vi "側推主程式(c58).vi"() -> ()   [LabVIEW 2021]
uses:
  <vilib>/Analysis/baseanly.llb/Mean (DBL).vi
  <vilib>/Analysis/NI_AALBase.lvlib
panel:
  out "Save A":bool
  out "Save 9":bool
  out "Save 7":bool
  out "A stop":bool
  out "A run":bool
  out "R stop":bool
  out "R run":bool
  out "AO stop":bool
  out "AO run":bool
  in  "Tab Control":T1(tab)
  in  "Tab Control 2":enum32{"循環加載", "線性加載", "定值加載"}(tab)
  out "AO Chart basic_cyc":dbl(graph)
  out "XY end":dbl=1.0
  out "basic end":dbl
  in  "AO stop\n(F時連續cyc)\n(T時停止AO)":bool
  out "t'(目前加載次數)":dbl
  out "T為完成加載":bool
  out "dt(目前歷時)":dbl
  out "duration":dbl
  in  "number of cyc":dbl
  out "AO Chart y_cyc":dbl(graph)
  out "AO Chart x_cyc":dbl(graph)
  in  "basic":dbl
  in  "cyc平移調整y":dbl
  in  "cyc震幅調整y":dbl
  in  "(basic+震幅)\ncyc平移調整x":dbl
  in  "cyc震幅調整x":dbl
  in  "fre(Hz)":dbl
  in  "milliseconds to (設定0)":u32
  in  "線性電壓斜率y":dbl
  in  "線性電壓斜率x":dbl
  out "線性加載 Chart":dynamicdata(graph)
  in  "線性加載初值 Y":dbl
  in  "線性加載初值 X":dbl
  in  "線性加載 basic":dbl
  out "非循環歷時 2":dbl
  out "線性加載\nbasic end":dbl
  in  "線性加載\n(F為連續)\n(T為停止)":bool
  out "XY end":dbl=1.0
  out "EP_X":dbl
  out "EP_Y":dbl
  out "EP_B":dbl
  out "非循環歷時":dbl
  out "定值加載\nbasic end":dbl
  out "XY end":dbl=1.0
  in  "定值加載\n(F為連續)\n(T為停止)":bool
  in  "定值加載 Y":dbl
  in  "定值加載 X":dbl
  in  "定值加載 basic":dbl
  out "定值加載 Chart":dynamicdata(graph)
  in  "線性加載\n(T為X加載)\n(F為Y加載)":bool
  in  "非循環加載\n(T為定值加載)\n(F為線性加載)":bool
  in  "循環加載\n(T為循環加載)\n(F為非循環加載)":bool
  in  "T為開始側推\nF為等待下一步指令\n(一開始先T)":bool
  out "Waveform Chart S7":dynamicdata(graph)
  in  "rate S7":dbl=1000.0
  in  "number of samples S7":i32=100
  out "Waveform Chart S9":dynamicdata(graph)
  in  "number of samples S9":i32=100
  in  "rate S9":dbl=1000.0
  in  "Enable S7":bool=TRUE caption="Enable"
  in  "Filename S7":path=path "test.lvm" caption="Filename"
  in  "Enable S9":bool=TRUE caption="Enable"
  in  "Filename S9":path=path "test.lvm" caption="Filename"
  in  "F 為\n開始 reading\n(AO is continue)":bool
  out "ACC紀錄中":bool
  out "Waveform Graph ACC":dynamicdata(graph)
  in  "number of samples":i32=2000
  in  "rate":dbl=20000.0
  in  "Enable":bool=TRUE
  in  "Filename":path=path "test.lvm"
  in  "Boolean\n(T為開始記讀)\n(F為停止記讀)\n(T後請手動調成F，避免重複執行)":bool
  out "Waveform Chart 角度cos_Y 3":dbl(graph)
  out "Waveform Chart LDT_X real":dynamicdata(graph)
  out "Waveform Chart load real 2":dynamicdata(graph)
  out "Waveform Chart 樁頭dis_X":dbl(graph)
  in  "LDT20係數":dbl
  in  "LDT20初值":dbl
  in  "LDT29係數":dbl
  in  "LDT29初值":dbl
  in  "LDT11初值":dbl
  in  "LDT11係數":dbl
  in  "LDT12係數":dbl
  in  "LDT12初值":dbl
  in  "PPT_B係數":dbl
  in  "PPT_B初值":dbl
  in  "PPT_C係數":dbl
  in  "PPT_C初值":dbl
  in  "PPT_E係數":dbl
  in  "PPT_E初值":dbl
  in  "PPT_F係數":dbl
  in  "PPT_F初值":dbl
  out "Waveform Chart PPT real":dynamicdata(graph)
  out "Waveform Chart load real":dynamicdata(graph)
  in  "load_X初值":dbl
  in  "load_Y初值":dbl
  in  "load_X係數":dbl
  in  "load_Y係數":dbl
  out "LDT20 real":dbl
  out "LDT29 real":dbl
  out "LDT12 real":dbl
  out "LDT11 real":dbl
  in  "LDT_X間距\n(cm)_3-4cm":dbl
  in  "LDT_Y間距\n(cm)_5.2cm":dbl
  out "LDT_Y斜率":dbl
  out "LDT_X斜率":dbl
  out "樁頭位移_X(cm)":dbl
  out "樁頭位移_Y(cm)":dbl
  in  "樁頭離\n下側LDT距_X\n(cm)":dbl
  in  "樁頭離\n下側LDT距_Y\n(cm)":dbl
  out "樁角度_Y_tan":dbl
  out "樁角度_X_tan":dbl
  out "Waveform Chart 樁頭dis_Y":dbl(graph)
  out "Waveform Chart 角度tan_Y":dbl(graph)
  out "Waveform Chart 角度tan_X":dbl(graph)
  out "樁角度_Y_cos":dbl
  out "Waveform Chart 角度cos_X":dbl(graph)
  out "樁角度_X_cos":dbl
  out "mean_load_Y":dbl format="%0.2f"
  out "mean_load_X":dbl format="%0.2f"
  out "Waveform Chart LDT_Y real 2":dynamicdata(graph)
  out "Waveform Chart LDT_Y real":dynamicdata(graph)
  out "Waveform Chart LDT_X real 2":dynamicdata(graph)
  # "AO"
  # "Read"
  # "ACC"
  # "資料擷取比\n電壓輸出快3s"
  # "循環"
  # "basic = XY\n完成反覆側推後\n側推力平衡"
  # "線性\n分X、Y向"
  # "定值"
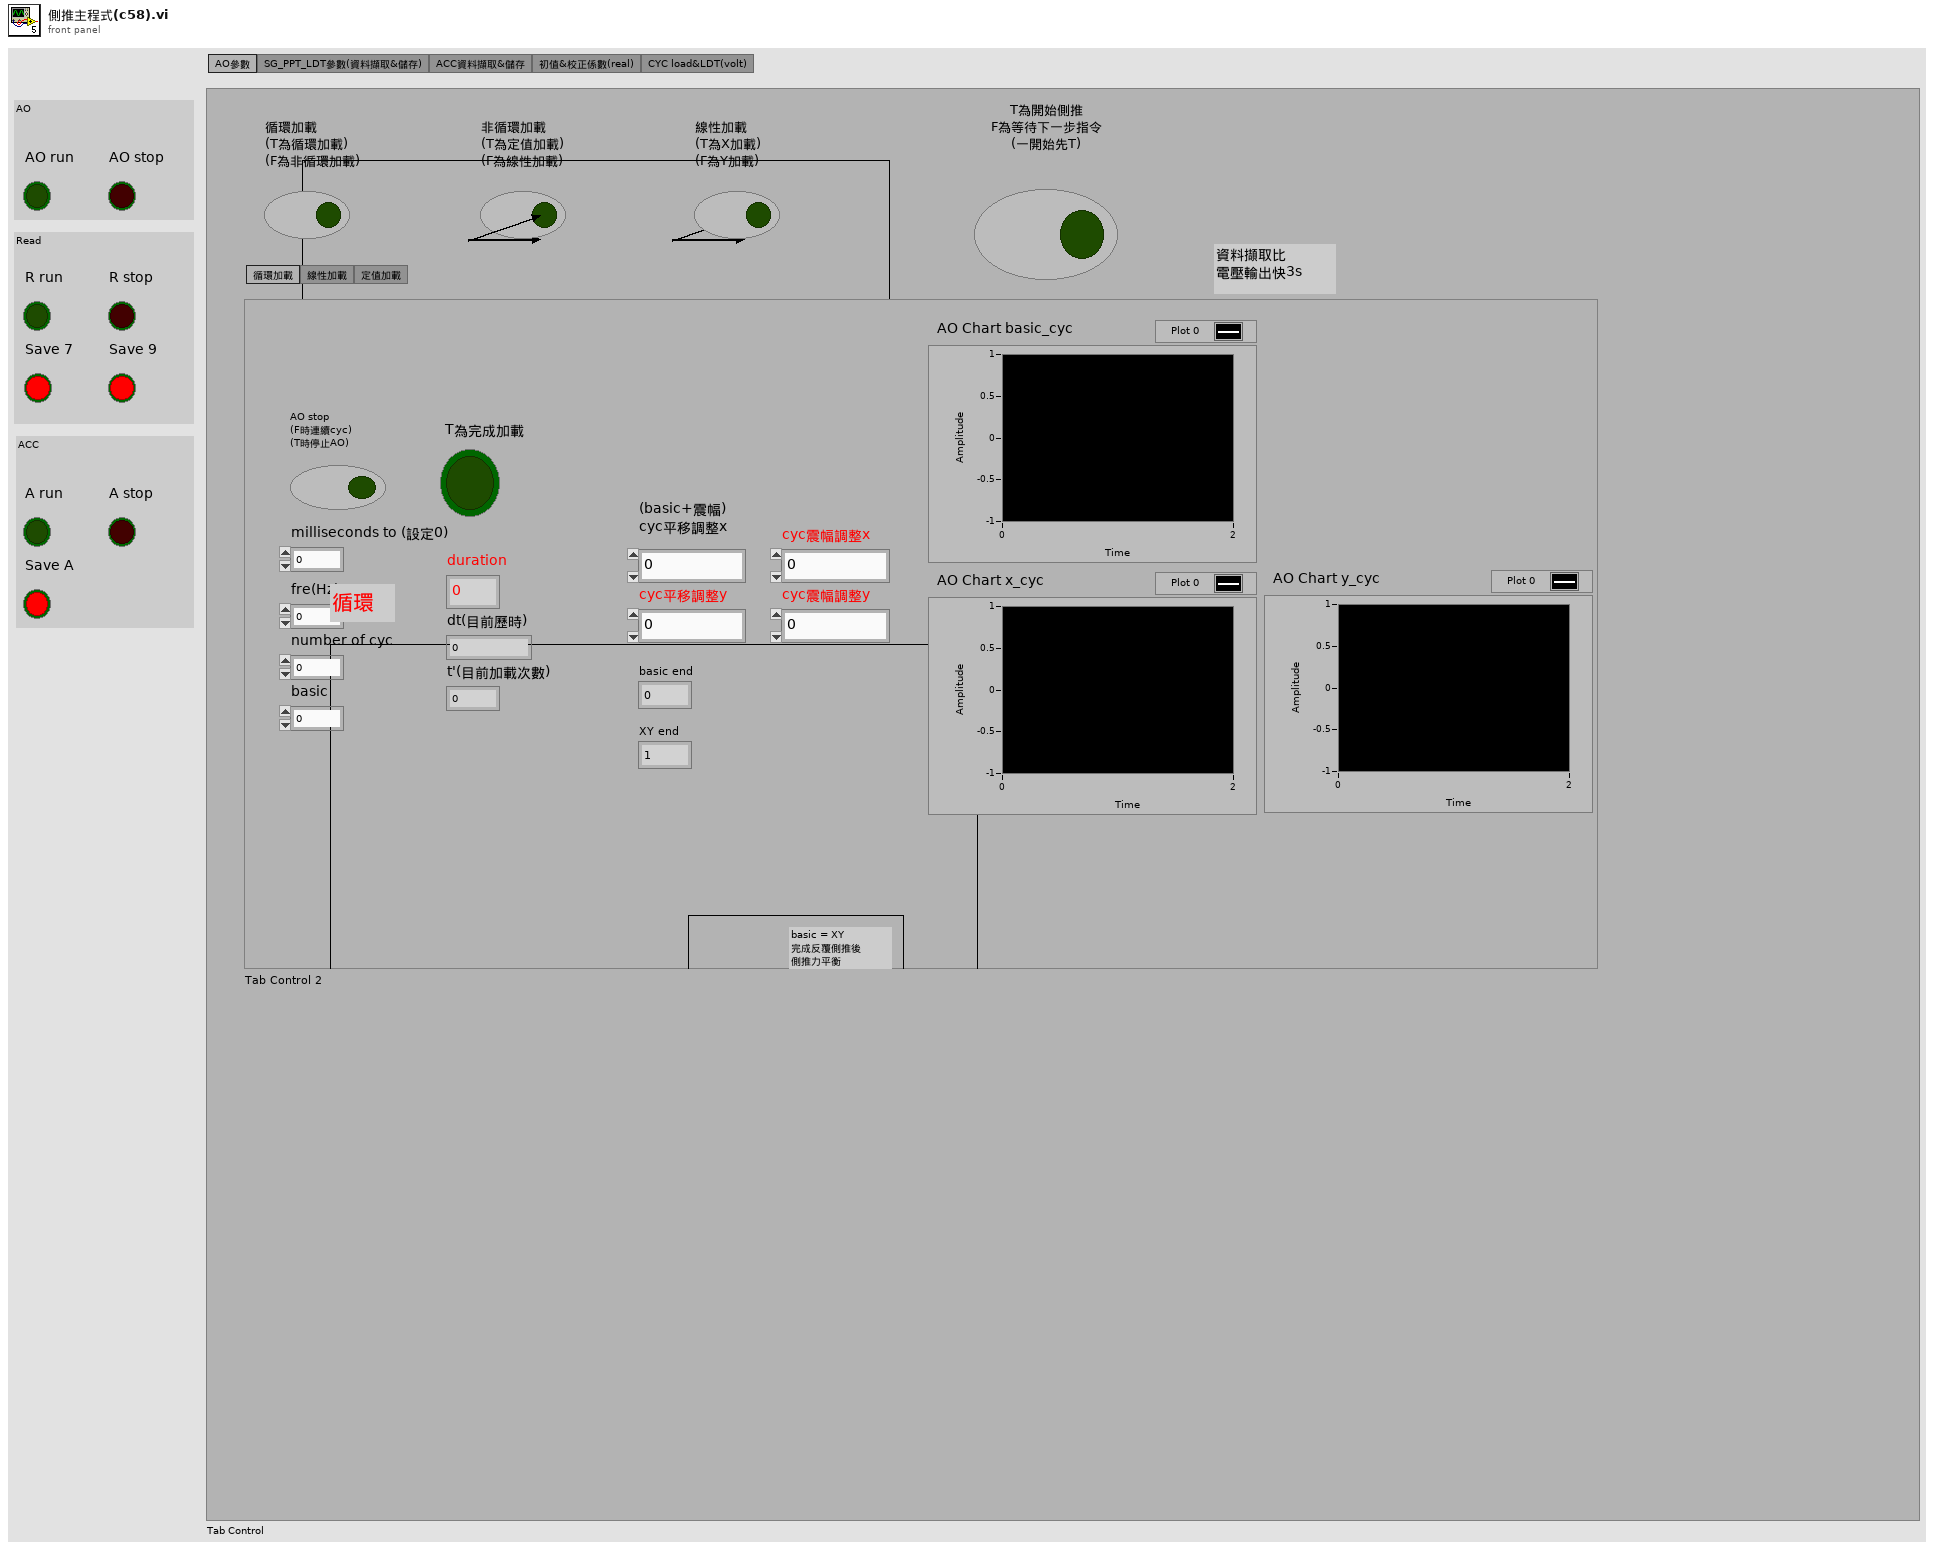
[diagram p1: front panel]
types:
  T1 = enum32{"AO參數", "SG_PPT_LDT參數(資料擷取&儲存)", "ACC資料擷取&儲存", "初值&校正係數(real)", "CYC load&LDT(volt)"}
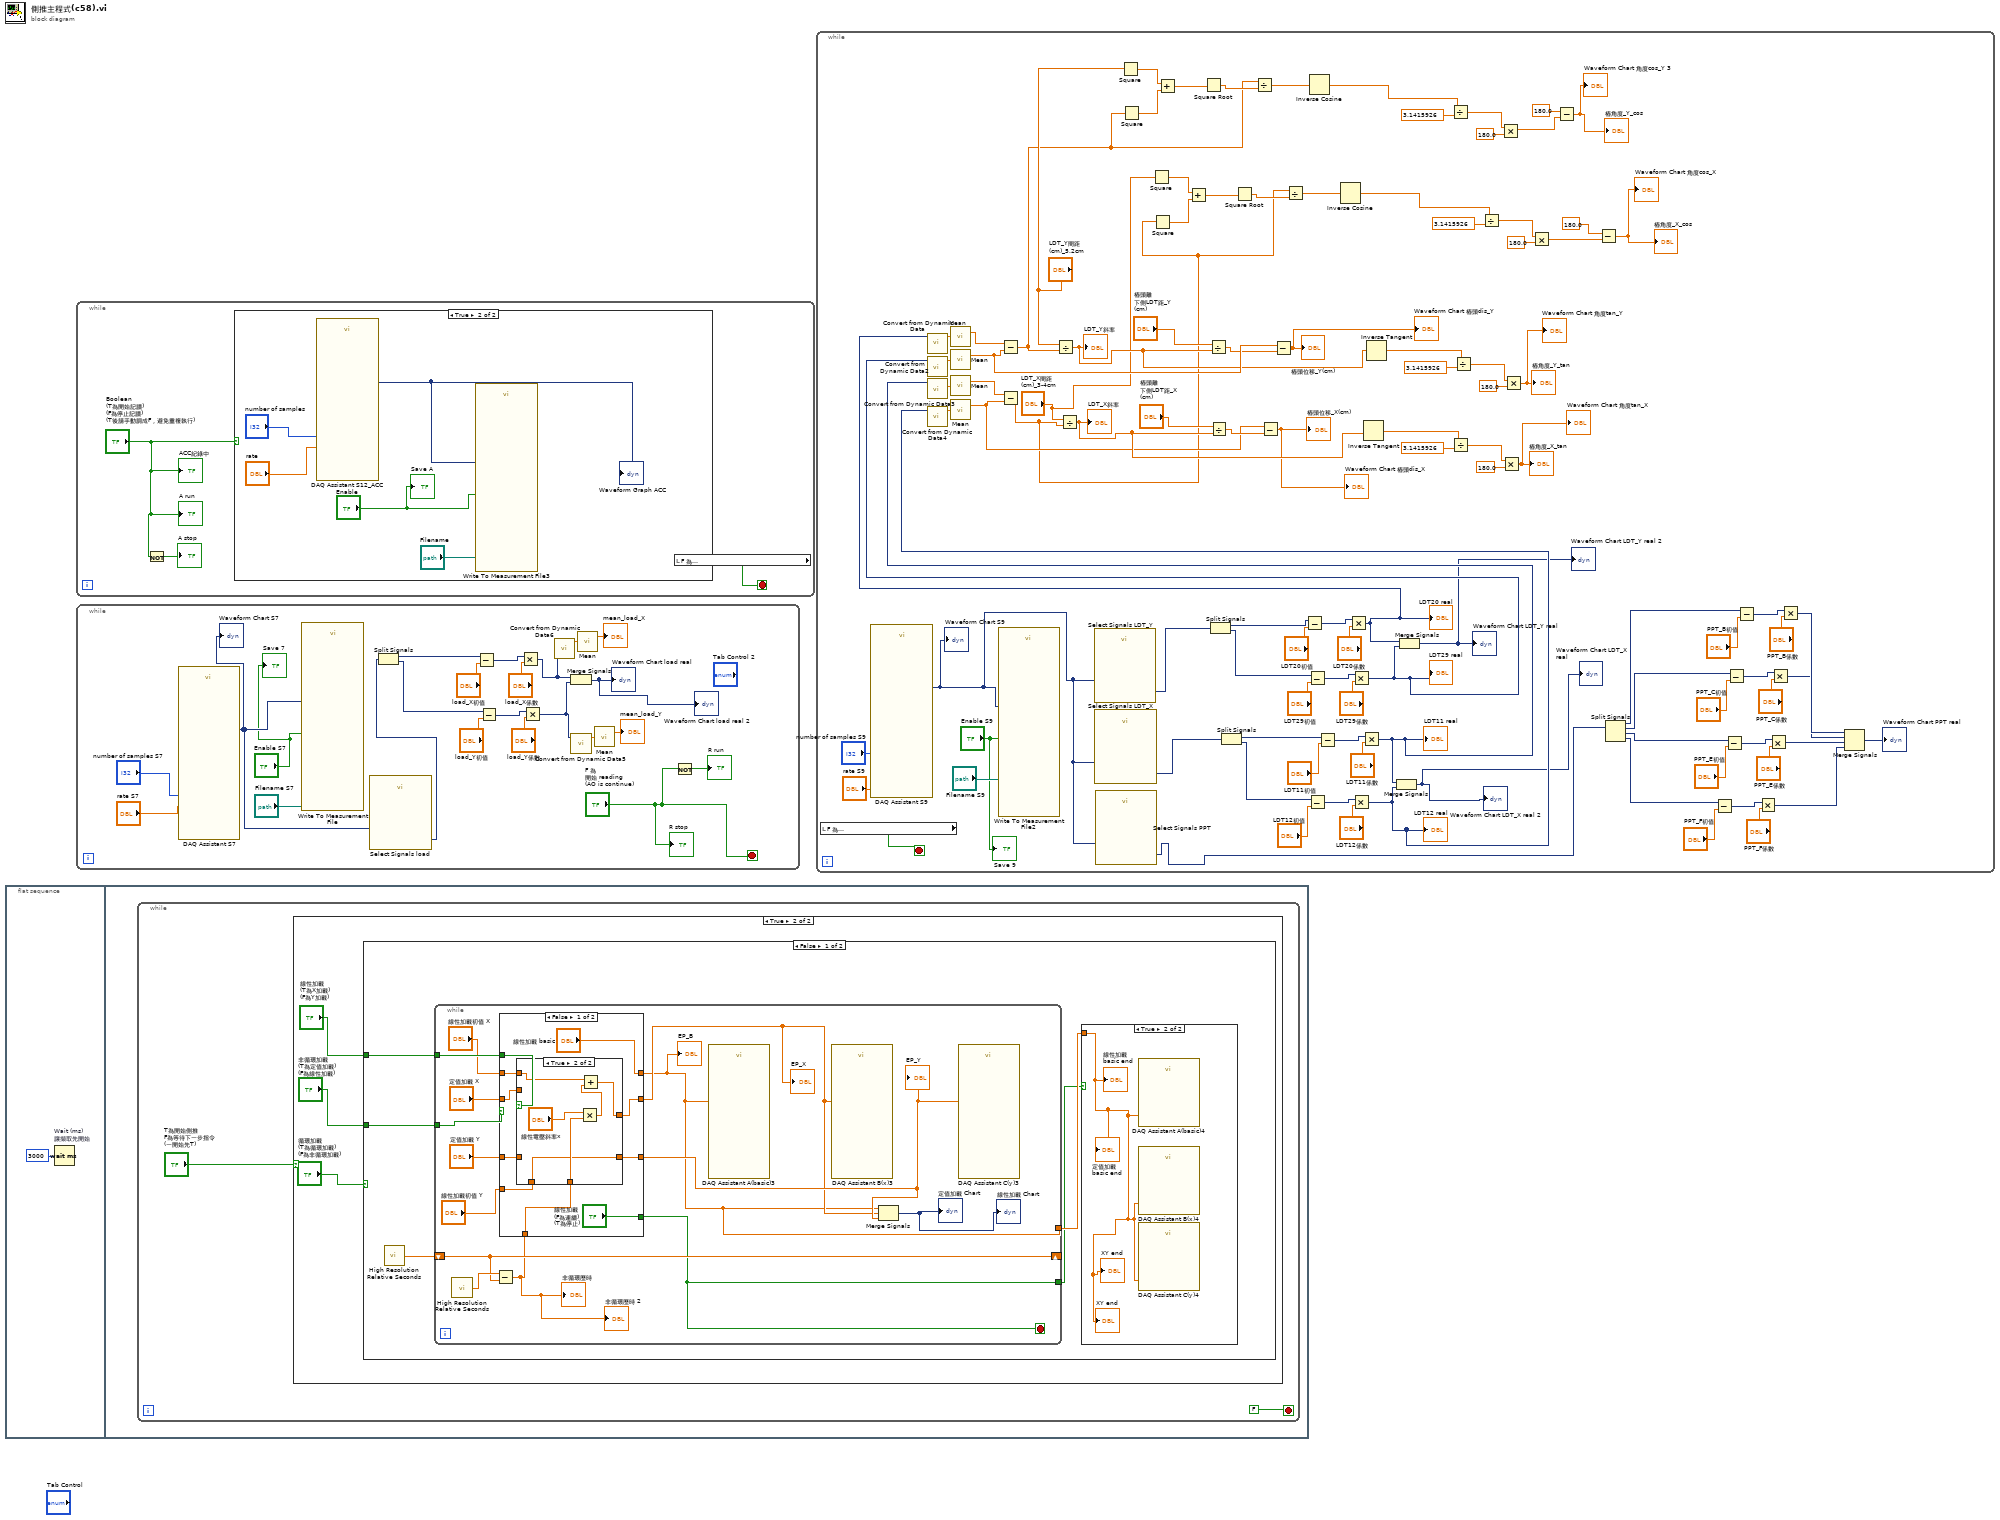
[diagram p0: block diagram]
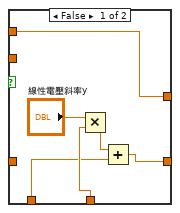
[diagram p5: hidden frame]
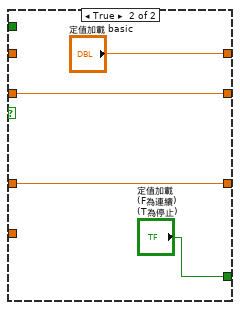
[diagram p6: hidden frame]
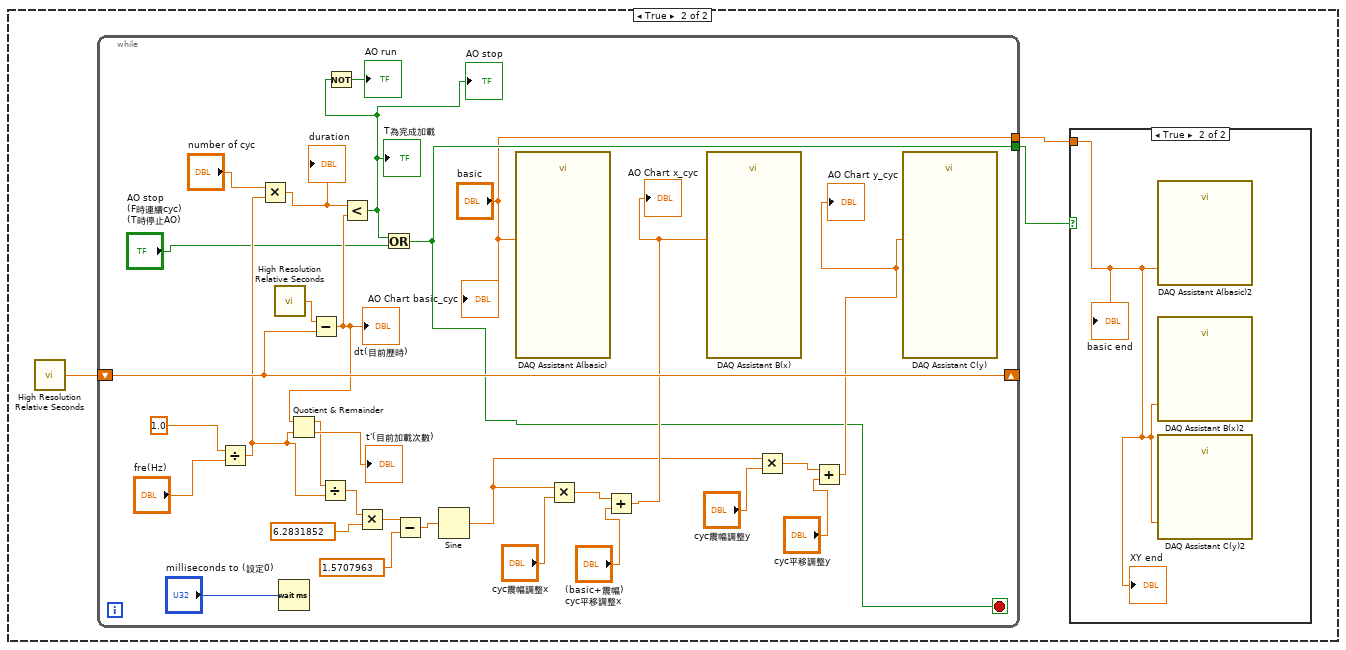
[diagram p7: hidden frame]
diagram:
  n1 = flat-sequence {
    frame #0 {
      n2 = Wait (ms) "Wait (ms)\n讓擷取先開始"(milliseconds to wait=u32 3000) -> ()  [unwired: 1 out]
    }
    frame #1 {
      n3 = while {
        stop <- FALSE stop-if-true
        n4 = case shown="True" "T為開始側推\nF為等待下一步指令\n(一開始先T)" {
          frame False {
          }
          frame True {
            n5 = case shown="False" "循環加載\n(T為循環加載)\n(F為非循環加載)" {
              tunnel: "非循環加載\n(T為定值加載)\n(F為線性加載)" -> [w8 _]
              tunnel: "線性加載\n(T為X加載)\n(F為Y加載)" -> [w7 _]
              frame False {
                n6 = call <vilib>:"High Resolution Relative Seconds.vi"() -> ("relative seconds"=w10:dbl)
                n7 = while {
                  tunnel: [w13] -> w11
                  shift-right: [w25] -> _
                  shift-left: w10 -> [w25]
                  tunnel: [w15] -> w9
                  tunnel: w8 -> [w24]
                  tunnel: w7 -> [w20]
                  stop <- w15 stop-if-true
                  n8 = call <vilib>:"High Resolution Relative Seconds.vi"() -> ("relative seconds"=w26:dbl)
                  n9 = Subtract(x=w26, y=w25) -> (x-y=w16:dbl)
                  "非循環歷時" <- w16
                  "非循環歷時 2" <- w16
                  n10 = case shown="False" w24 {
                    tunnel: "定值加載 X" -> [w31 w52]
                    tunnel: [w33 w52] -> w14
                    tunnel: "定值加載 Y" -> [w34 w51]
                    tunnel: [w32 w51] -> w21
                    tunnel: w16 -> [w36 _]
                    tunnel: w20 -> [w35 _]
                    tunnel: "線性加載初值 X" -> [w30 _]
                    tunnel: "線性加載初值 Y" -> [w29 _]
                    tunnel: ["線性加載 basic" "定值加載 basic"] -> w13
                    tunnel: ["線性加載\n(F為連續)\n(T為停止)" "定值加載\n(F為連續)\n(T為停止)"] -> w15
                    frame False {
                      n11 = case shown="True" w35 {
                        tunnel: w36 -> [w41 w47]
                        tunnel: [w40 w43] -> w33
                        tunnel: w34 -> [_ _]
                        tunnel: [w37 w46] -> w32
                        tunnel: w31 -> [_ _]
                        tunnel: w30 -> [w40 w45]
                        tunnel: w29 -> [w38 w46]
                        frame False {
                          n12 = Multiply(x="線性電壓斜率y", y=w41) -> (x*y=w39:dbl)
                          n13 = Add(x=w39, y=w38) -> (x+y=w37:dbl)
                        }
                        frame True {
                          n14 = Multiply(x="線性電壓斜率x", y=w47) -> (x*y=w44:dbl)
                          n15 = Add(x=w45, y=w44) -> (x+y=w43:dbl)
                        }
                      }
                    }
                    frame True {
                    }
                  }
                  "EP_Y" <- w21
                  "EP_X" <- w14
                  "EP_B" <- w13
                  n16 = call "DAQ Assistant A(basic)3"("data"=w13) -> ()  [unwired: 17 in, 2 out]
                  n17 = call "DAQ Assistant B(x)3"("data"=w14) -> ()  [unwired: 17 in, 2 out]
                  n18 = Merge Signals(w13, w14, w21) -> (→"定值加載 Chart" →"線性加載 Chart":dynamicdata)
                  n19 = call "DAQ Assistant C(y)3"("data"=w21) -> ()  [unwired: 17 in, 2 out]
                }
                n20 = case shown="True" w9 {
                  tunnel: w11 -> [_ w12]
                  frame False {
                  }
                  frame True {
                    n21 = call "DAQ Assistant A(basic)4"("data"=w12) -> ()  [unwired: 17 in, 2 out]
                    n22 = call "DAQ Assistant B(x)4"("data"=w12) -> ()  [unwired: 17 in, 2 out]
                    n23 = call "DAQ Assistant C(y)4"("data"=w12) -> ()  [unwired: 17 in, 2 out]
                    "定值加載\nbasic end" <- w12
                    "XY end" <- w12
                    "線性加載\nbasic end" <- w12
                    "XY end" <- w12
                  }
                }
              }
              frame True {
                n24 = call <vilib>:"High Resolution Relative Seconds.vi"() -> ("relative seconds"=w55:dbl)
                n25 = while {
                  shift-right: [w85] -> _
                  shift-left: w55 -> [w85]
                  tunnel: [w64] -> w54
                  tunnel: ["basic"] -> w53
                  stop <- w64 stop-if-true
                  n26 = Divide(x=1.0, y="fre(Hz)") -> (x/y=w68:dbl)
                  n27 = Multiply(x="number of cyc", y=w68) -> (x*y=w67:dbl)
                  "duration" <- w67
                  n28 = call <vilib>:"High Resolution Relative Seconds.vi"() -> ("relative seconds"=w86:dbl)
                  n29 = Wait (ms)(milliseconds to wait="milliseconds to (設定0)") -> ()  [unwired: 1 out]
                  n30 = Subtract(x=w86, y=w85) -> (x-y=w66:dbl)
                  "dt(目前歷時)" <- w66
                  n31 = Quotient & Remainder(x=w66, y=w68) -> (x-y*floor(x/y)=w81:dbl, floor(x/y)=→"t'(目前加載次數)":dbl)
                  n32 = Divide(x=w81, y=w68) -> (x/y=w78:dbl)
                  n33 = Less?(x=w67, y=w66) -> (x < y?=w58:bool)
                  "T為完成加載" <- w58
                  "AO stop" <- w58
                  n34 = Not(x=w58) -> (.not. x?=→"AO run":bool)
                  n35 = Multiply(x=w78, y=6.2831852) -> (x*y=w61:dbl)
                  n36 = Or(x=w58, y="AO stop\n(F時連續cyc)\n(T時停止AO)") -> (x .or. y?=w64:bool)
                  n37 = Subtract(x=w61, y=1.5707963) -> (x-y=w60:dbl)
                  n38 = Sine(x=w60) -> (sin(x)=w59:dbl)
                  n39 = call "DAQ Assistant A(basic)"("data"="basic") -> ()  [unwired: 17 in, 2 out]
                  n40 = Multiply(x=w59, y="cyc震幅調整x") -> (x*y=w76:dbl)
                  n41 = Add(x=w76, y="(basic+震幅)\ncyc平移調整x") -> (x+y=w71:dbl)
                  "AO Chart x_cyc" <- w71
                  n42 = call "DAQ Assistant B(x)"("data"=w71) -> ()  [unwired: 17 in, 2 out]
                  n43 = Multiply(x=w59, y="cyc震幅調整y") -> (x*y=w73:dbl)
                  n44 = Add(x=w73, y="cyc平移調整y") -> (x+y=w70:dbl)
                  "AO Chart y_cyc" <- w70
                  n45 = call "DAQ Assistant C(y)"("data"=w70) -> ()  [unwired: 17 in, 2 out]
                  "AO Chart basic_cyc" <- "basic"
                }
                n46 = case shown="True" w54 {
                  tunnel: w53 -> [_ w56]
                  frame False {
                  }
                  frame True {
                    n47 = call "DAQ Assistant A(basic)2"("data"=w56) -> ()  [unwired: 17 in, 2 out]
                    n48 = call "DAQ Assistant B(x)2"("data"=w56) -> ()  [unwired: 17 in, 2 out]
                    n49 = call "DAQ Assistant C(y)2"("data"=w56) -> ()  [unwired: 17 in, 2 out]
                    "basic end" <- w56
                    "XY end" <- w56
                  }
                }
              }
            }
          }
        }
      }
    }
  }
  n50 = while {
    stop <- w89 stop-if-true
    n51 = Not(x="Boolean\n(T為開始記讀)\n(F為停止記讀)\n(T後請手動調成F，避免重複執行)") -> (.not. x?=→"A stop":bool)
    n52 = case shown="True" "Boolean\n(T為開始記讀)\n(F為停止記讀)\n(T後請手動調成F，避免重複執行)" {
      frame False {
      }
      frame True {
        n53 = call "DAQ Assistant S12_ACC"("rate"="rate", "number of samples"="number of samples") -> ("data"=w92:dynamicdata)  [unwired: 15 in, 2 out]
        "Waveform Graph ACC" <- w92
        n54 = call "Write To Measurement File3"("Signals"=w92, "Enable"="Enable", "Filename"="Filename") -> ()  [unwired: 14 in, 3 out]
        "Save A" <- "Enable"
      }
    }
    n55 = local read "F 為\n開始 reading\n(AO is continue)"() -> (w89:bool)
    "ACC紀錄中" <- "Boolean\n(T為開始記讀)\n(F為停止記讀)\n(T後請手動調成F，避免重複執行)"
    "A run" <- "Boolean\n(T為開始記讀)\n(F為停止記讀)\n(T後請手動調成F，避免重複執行)"
  }
  n56 = while {
    stop <- "F 為\n開始 reading\n(AO is continue)" stop-if-true
    n57 = call "DAQ Assistant S7"("rate"="rate S7", "number of samples"="number of samples S7") -> ("data"=w105:dynamicdata)  [unwired: 14 in, 3 out]
    "Waveform Chart S7" <- w105
    n58 = call "Write To Measurement File"("Signals"=w105, "Enable"="Enable S7", "Filename"="Filename S7") -> ()  [unwired: 14 in, 3 out]
    n59 = call "Select Signals load"("Signals"=w105) -> ("Signal Out"=w108:dynamicdata)  [unwired: 9 in, 1 out]
    n60 = Split Signals(w108) -> (w107:dynamicdata, w106:dynamicdata)  [unwired: 2 in]
    n61 = Subtract(x=w107, y="load_X初值") -> (x-y=w114:dynamicdata)
    n62 = Subtract(x=w106, y="load_Y初值") -> (x-y=w111:dynamicdata)
    n63 = Multiply(x=w114, y="load_X係數") -> (x*y=w100:dynamicdata)
    n64 = Multiply(x=w111, y="load_Y係數") -> (x*y=w104:dynamicdata)
    n65 = call "Convert from Dynamic Data6"("Dynamic Data Type"=w100) -> ("Array"=w99:dbl[])  [unwired: 3 in]
    n66 = Merge Signals(w100, w104) -> (→"Waveform Chart load real" →"Waveform Chart load real 2":dynamicdata)
    n67 = call "Convert from Dynamic Data5"("Dynamic Data Type"=w104) -> ("Array"=w103:dbl[])  [unwired: 3 in]
    n68 = call-poly <vilib>:"Mean.vi"("X"=w99) -> ("mean"=→"mean_load_X":dbl)  [unwired: 1 out]
    n69 = call-poly <vilib>:"Mean.vi"("X"=w103) -> ("mean"=→"mean_load_Y":dbl)  [unwired: 1 out]
    n70 = Not(x="F 為\n開始 reading\n(AO is continue)") -> (.not. x?=→"R run":bool)
    "R stop" <- "F 為\n開始 reading\n(AO is continue)"
    "Save 7" <- "Enable S7"
  }
  n71 = while {
    stop <- w127 stop-if-true
    n72 = local read "F 為\n開始 reading\n(AO is continue)"() -> (w127:bool)
    n73 = call "DAQ Assistant S9"("rate"="rate S9", "number of samples"="number of samples S9") -> ("data"=w220:dynamicdata)  [unwired: 14 in, 3 out]
    "Waveform Chart S9" <- w220
    n74 = call "Write To Measurement File2"("Signals"=w220, "Enable"="Enable S9", "Filename"="Filename S9") -> ()  [unwired: 14 in, 3 out]
    n75 = call "Select Signals LDT_Y"("Signals"=w220) -> ("Signal Out"=w219:dynamicdata)  [unwired: 9 in, 1 out]
    n76 = call "Select Signals LDT_X"("Signals"=w220) -> ("Signal Out"=w208:dynamicdata)  [unwired: 9 in, 1 out]
    n77 = call "Select Signals PPT"("Signals"=w220) -> ("Signal Out"=w184:dynamicdata)  [unwired: 9 in, 1 out]
    n78 = Square(x="LDT_Y間距\n(cm)_5.2cm") -> (x^2=w149:dbl)
    n79 = Square(x="LDT_X間距\n(cm)_3-4cm") -> (x^2=w138:dbl)
    n80 = Split Signals(w219) -> (w216:dynamicdata, w211:dynamicdata)  [unwired: 2 in]
    n81 = Split Signals(w208) -> (w206:dynamicdata, w202:dynamicdata)  [unwired: 2 in]
    n82 = Subtract(x=w216, y="LDT20初值") -> (x-y=w218:dynamicdata)
    n83 = Subtract(x=w211, y="LDT29初值") -> (x-y=w214:dynamicdata)
    n84 = Subtract(x=w202, y="LDT12初值") -> (x-y=w205:dynamicdata)
    n85 = Subtract(x=w206, y="LDT11初值") -> (x-y=w210:dynamicdata)
    n86 = Multiply(x=w218, y="LDT20係數") -> (x*y=w179:dynamicdata)
    "LDT20 real" <- w179
    n87 = call "Convert from Dynamic Data"("Dynamic Data Type"=w179) -> ("Array"=w178:dbl[])  [unwired: 3 in]
    n88 = call-poly <vilib>:"Mean.vi"("X"=w178) -> ("mean"=w170:dbl)  [unwired: 1 out]
    n89 = Multiply(x=w214, y="LDT29係數") -> (x*y=w177:dynamicdata)
    "LDT29 real" <- w177
    n90 = call "Convert from Dynamic Data2"("Dynamic Data Type"=w177) -> ("Array"=w176:dbl[])  [unwired: 3 in]
    n91 = call-poly <vilib>:"Mean.vi"("X"=w176) -> ("mean"=w167:dbl)  [unwired: 1 out]
    n92 = Subtract(x=w170, y=w167) -> (x-y=w139:dbl)
    n93 = Divide(x="LDT_Y間距\n(cm)_5.2cm", y=w139) -> (x/y=w160:dbl)
    "LDT_Y斜率" <- w160
    n94 = Square(x=w139) -> (x^2=w148:dbl)
    n95 = Add(x=w149, y=w148) -> (x+y=w147:dbl)
    n96 = Square Root(x=w147) -> (sqrt(x)=w146:dbl)
    n97 = Divide(x="樁頭離\n下側LDT距_Y\n(cm)", y=w160) -> (x/y=w166:dbl)
    n98 = Divide(x=w139, y=w146) -> (x/y=w144:dbl)
    n99 = Subtract(x=w167, y=w166) -> (x-y=→"樁頭位移_Y(cm)" →"Waveform Chart 樁頭dis_Y":dbl)
    n100 = Inverse Cosine(1:w144) -> (0:w140:dbl)
    n101 = Multiply(x=w205, y="LDT12係數") -> (x*y=w173:dynamicdata)
    "LDT12 real" <- w173
    n102 = call "Convert from Dynamic Data4"("Dynamic Data Type"=w173) -> ("Array"=w172:dbl[])  [unwired: 3 in]
    n103 = call-poly <vilib>:"Mean.vi"("X"=w172) -> ("mean"=w151:dbl)  [unwired: 1 out]
    n104 = Multiply(x=w210, y="LDT11係數") -> (x*y=w175:dynamicdata)
    "LDT11 real" <- w175
    n105 = call "Convert from Dynamic Data3"("Dynamic Data Type"=w175) -> ("Array"=w174:dbl[])  [unwired: 3 in]
    n106 = call-poly <vilib>:"Mean.vi"("X"=w174) -> ("mean"=w171:dbl)  [unwired: 1 out]
    n107 = Subtract(x=w171, y=w151) -> (x-y=w128:dbl)
    n108 = Divide(x="LDT_X間距\n(cm)_3-4cm", y=w128) -> (x/y=w155:dbl)
    "LDT_X斜率" <- w155
    n109 = Square(x=w128) -> (x^2=w137:dbl)
    n110 = Add(x=w138, y=w137) -> (x+y=w136:dbl)
    n111 = Divide(x="樁頭離\n下側LDT距_X\n(cm)", y=w155) -> (x/y=w165:dbl)
    n112 = Square Root(x=w136) -> (sqrt(x)=w135:dbl)
    n113 = Subtract(x=w151, y=w165) -> (x-y=→"樁頭位移_X(cm)" →"Waveform Chart 樁頭dis_X":dbl)
    n114 = Divide(x=w128, y=w135) -> (x/y=w134:dbl)
    n115 = Inverse Cosine(1:w134) -> (0:w130:dbl)
    n116 = Inverse Tangent(1:w155) -> (0:w157:dbl)
    n117 = Inverse Tangent(1:w160) -> (0:w162:dbl)
    n118 = Merge Signals(w175, w173) -> (→"Waveform Chart LDT_X real 2" →"Waveform Chart LDT_X real":dynamicdata)
    n119 = Merge Signals(w179, w177) -> (→"Waveform Chart LDT_Y real" →"Waveform Chart LDT_Y real 2":dynamicdata)
    n120 = Divide(x=w140, y=3.1415926) -> (x/y=w141:dbl)
    n121 = Divide(x=w157, y=3.1415926) -> (x/y=w156:dbl)
    n122 = Divide(x=w162, y=3.1415926) -> (x/y=w161:dbl)
    n123 = Divide(x=w130, y=3.1415926) -> (x/y=w131:dbl)
    n124 = Multiply(x=w141, y=180.0) -> (x*y=w122:dbl)
    n125 = Multiply(x=w156, y=180.0) -> (x*y=→"樁角度_X_tan" →"Waveform Chart 角度tan_X":dbl)
    n126 = Multiply(x=w161, y=180.0) -> (x*y=→"樁角度_Y_tan" →"Waveform Chart 角度tan_Y":dbl)
    n127 = Multiply(x=w131, y=180.0) -> (x*y=w121:dbl)
    n128 = Subtract(x=180.0, y=w122) -> (x-y=→"樁角度_Y_cos" →"Waveform Chart 角度cos_Y 3":dbl)
    n129 = Subtract(x=180.0, y=w121) -> (x-y=→"樁角度_X_cos" →"Waveform Chart 角度cos_X":dbl)
    n130 = Split Signals(w184) -> (w183:dynamicdata, w182:dynamicdata, w181:dynamicdata, w180:dynamicdata)  [unwired: 4 in]
    n131 = Subtract(x=w180, y="PPT_F初值") -> (x-y=w190:dynamicdata)
    n132 = Subtract(x=w181, y="PPT_E初值") -> (x-y=w193:dynamicdata)
    n133 = Subtract(x=w182, y="PPT_C初值") -> (x-y=w198:dynamicdata)
    n134 = Subtract(x=w183, y="PPT_B初值") -> (x-y=w201:dynamicdata)
    n135 = Multiply(x=w190, y="PPT_F係數") -> (x*y=w186:dynamicdata)
    n136 = Multiply(x=w193, y="PPT_E係數") -> (x*y=w187:dynamicdata)
    n137 = Multiply(x=w198, y="PPT_C係數") -> (x*y=w194:dynamicdata)
    n138 = Multiply(x=w201, y="PPT_B係數") -> (x*y=w195:dynamicdata)
    n139 = Merge Signals(w195, w194, w187, w186) -> (→"Waveform Chart PPT real":dynamicdata)
    "Save 9" <- "Enable S9"
  }
